vi "ToolBarButtonDraw_ZoomWH.vi"(6 "Color":u32(colorbox), 10 "rect":T1, 11 "Pict IN":picture) -> (3 "Pict OUT":picture)   [LabVIEW 2020, in "Gviewer.lvclass"]
doc: "Draw Zoom Horizontal button content"
uses:
  Gviewer.lvclass
  <vilib>/picture/picture.llb/imagedata.ctl
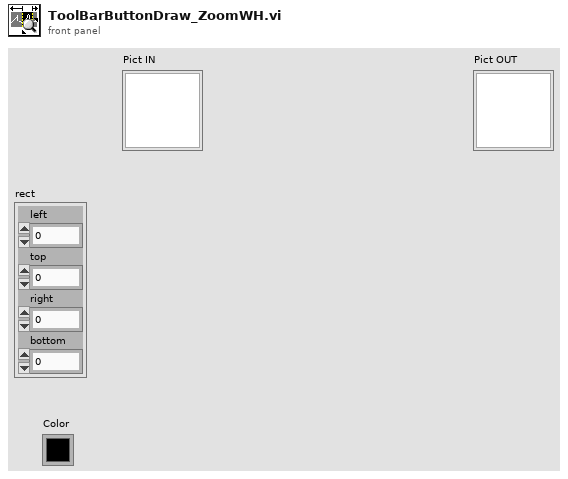
[diagram p1: front panel]
types:
  T1 = cluster{"left":i16, "top":i16, "right":i16, "bottom":i16}
  T2 = typedef "imagedata.ctl" = cluster{"image type":i32, "image depth":i32, "image":u8[], "mask":u8[], "colors":u32[], "Rectangle":cluster{"left":i16, "top":i16, "right":i16, "bottom":i16}}
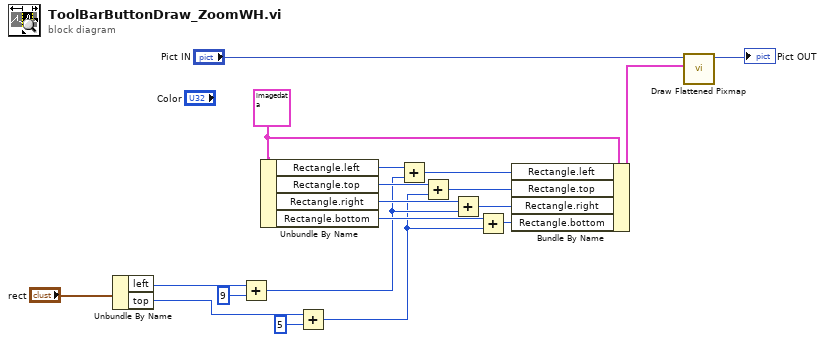
[diagram p0: block diagram]
diagram:
  w1 = T2 {"image type"=0, "image depth"=24, "image"=array[1170 elements], "mask"=[], "colors"=[], "Rectangle"={"left"=0, "top"=0, "right"=26, "bottom"=15}} ("image data")
  n1 = Unbundle By Name("rect") -> ("left"=w12:i16, "top"=w10:i16)
  n2 = Add(x=w12, y=i16 9) -> (x+y=w11:i16)
  n3 = Unbundle By Name(w1) -> ("Rectangle.left"=w16:i16, "Rectangle.top"=w15:i16, "Rectangle.right"=w14:i16, "Rectangle.bottom"=w13:i16)
  n4 = Add(x=w10, y=i16 5) -> (x+y=w9:i16)
  n5 = Add(x=w16, y=w11) -> (x+y=w5:i16)
  n6 = Add(x=w15, y=w9) -> (x+y=w6:i16)
  n7 = Add(x=w14, y=w11) -> (x+y=w7:i16)
  n8 = Add(x=w13, y=w9) -> (x+y=w8:i16)
  n9 = Bundle By Name(cluster=w1, "Rectangle.left"=w5, "Rectangle.top"=w6, "Rectangle.right"=w7, "Rectangle.bottom"=w8) -> (w4:T2)
  n10 = call <vilib>:"Draw Flattened Pixmap.vi"("image data"=w4, "picture"="Pict IN") -> ("new picture"=→"Pict OUT":picture)  [unwired: 7 in]
